vi "Construct.vi"(8 "error in":errorcluster, 9 "status error channel data references":T2 {"specific errors"."timeout" format="%.0x"; "specific errors"."bit timing" format="%.0x"; "specific errors"."long word" format="%.0x"; "specific errors"."parity" format="%.0x"; "specific errors"."gap" format="%.0x"; "receiving" format="%.0x"}, 10 "RT hardware channels":T3[](array[typedef]) {"labels settings for RT"."Label Timestamp Channel Data Reference" format="%.0x"; "labels settings for RT"."Word Initial Raw Value" format="%032.0f"; "labels settings for RT"."Label Disable/Trigger Channel Reference" format="%.0x"; "labels settings for RT"."parameter driver data"."Tx parameter refs" format="%.0x"; "labels settings for RT"."parameter driver data"."Rx block data refs"."Data Reference" format="%.0x"; "labels settings for RT"."SDI" format="%02b"; "labels settings for RT"."label" format="%.0o"}, 11 "ID":string) -> (0 "error out":errorcluster, 3 "Ballard ARINC-429 Rx Execution Unit":refnum<class "Ballard ARINC-429 Rx Execution Unit.lvclass">)   [LabVIEW 2020, in "Ballard ARINC 429 Engine.lvlib" / "Implementation.lvlib" / "Ballard ARINC-429 Rx Execution Unit.lvclass"]
uses:
  Ballard ARINC-429 Rx Execution Unit.lvclass
  Shared/RT Hardware Channel Settings.ctl
  Shared/RT Label Settings.ctl
  Shared/Label.ctl
  Shared/RT Parameters.ctl
  Shared/Parameter Definition.ctl
  Encoding and Decoding/Encoding.ctl
  <vilib>/NI VeriStand/Custom Device API/Block Data Reference.ctl
  <vilib>/NI VeriStand/Custom Device API/Data Reference.ctl
  <vilib>/NI VeriStand/Custom Device API/Custom Device Item Ref.ctl
  Shared/Transfer Type.ctl
  C:/Git/niveristand-ballard-arinc429-custom-device/Source/Custom Device Support/Engine/Implementation/Ballard ARINC-429 Execution Unit/Ballard ARINC-429 Execution Unit.lvclass
  Ballard ARINC-429 Execution Unit/Ballard ARINC-429 Execution Unit.lvclass/Ballard ARINC-429 Execution Unit.ctl
  Ballard ARINC-429 Rx Execution Unit.lvclass/Ballard ARINC-429 Rx Execution Unit.ctl
  Ballard ARINC-429 Execution Unit/Ballard ARINC-429 Execution Unit.lvclass
  C:/Git/niveristand-ballard-arinc429-custom-device/Source/Custom Device Support/Engine/Interfaces/Execution Unit/Execution Unit.lvclass
  C:/Git/niveristand-ballard-arinc429-custom-device/Source/Custom Device Support/Engine/Implementation/Ballard ARINC-429 Rx Execution Unit/Ballard ARINC-429 Rx Execution Unit.lvclass
  Encoding and Decoding/Encoding and Decoding.lvlib
  <vilib>/NI VeriStand/Custom Device API/Custom Device API.lvlib
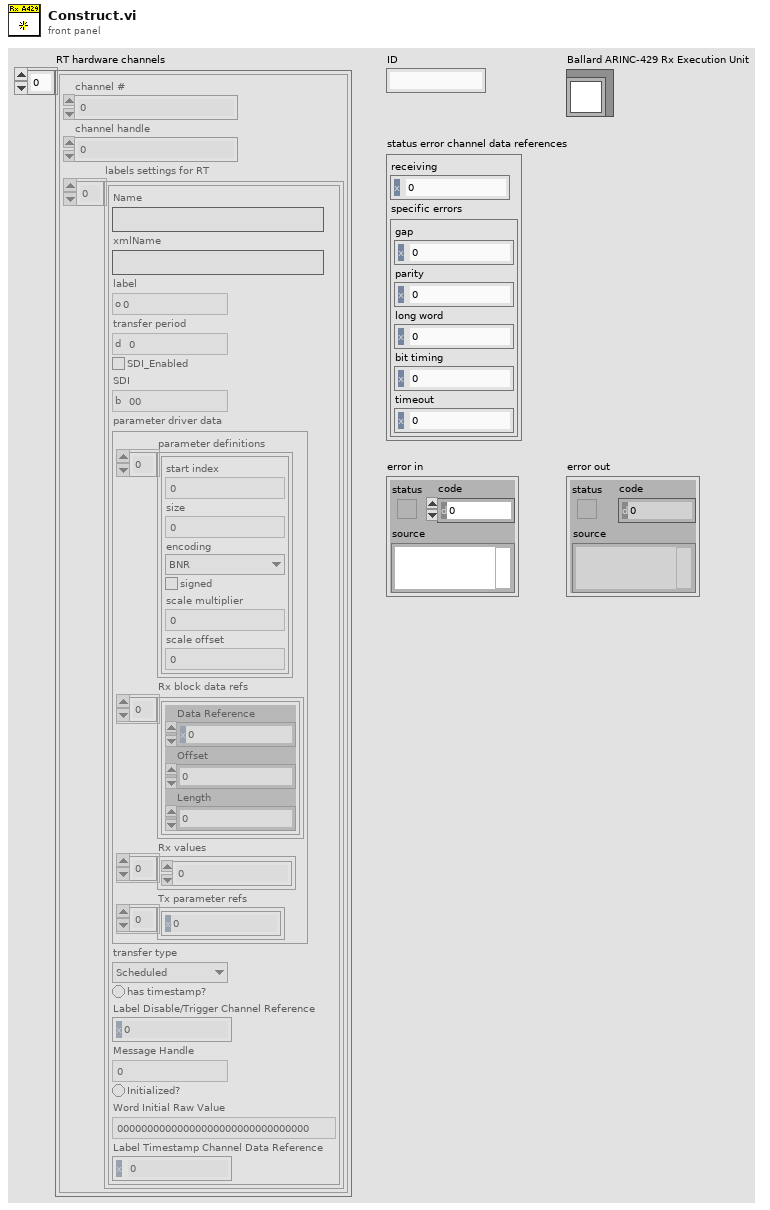
[diagram p1: front panel]
types:
  T1 = typedef "Custom Device API.lvlib/Data Reference.ctl" = i32
  T2 = cluster{"receiving":T1, "specific errors":cluster{"gap":T1, "parity":T1, "long word ":T1, "bit timing":T1, "timeout":T1}}
  T3 = typedef "RT Hardware Channel Settings.ctl" = cluster{"channel #":u16, "channel handle":u64, "labels settings for RT":T4[]}
  T4 = typedef "RT Label Settings.ctl" = cluster{"Name":string, "xmlName":string, "label":T5, "transfer period":u32, "SDI_Enabled":bool, "SDI":u8, "parameter driver data":T6, "transfer type":T11, "has timestamp?":bool, "Label Disable/Trigger Channel Reference":T10, "Message Handle":u64, "Initialized?":bool, "Word Initial Raw Value":u32, "Label Timestamp Channel Data Reference":T1}
  T5 = typedef "Label.ctl" = u8
  T6 = typedef "RT Parameters.ctl" = cluster{"parameter definitions":T7[], "Rx block data refs":T9[], "Rx values":dbl[], "Tx parameter refs":T10[]}
  T7 = typedef "Parameter Definition.ctl" = cluster{"start index":i32, "size":i32, "encoding":T8, "signed":bool, "scale multiplier":dbl, "scale offset":dbl}
  T8 = typedef "Encoding and Decoding.lvlib/Encoding.ctl" = enum16{"BNR", "BCD", "Discrete"}
  T9 = typedef "Custom Device API.lvlib/Block Data Reference.ctl" = cluster{"Data Reference":T1, "Offset":u64, "Length":u64}
  T10 = typedef "Custom Device API.lvlib/Custom Device Item Ref.ctl" = u64
  T11 = typedef "Transfer Type.ctl" = enum16{"Scheduled", "Acyclic", "Block", "Strobe"}
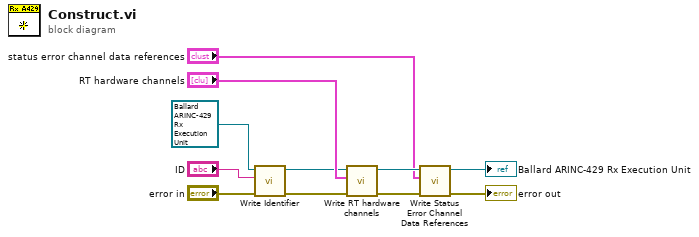
[diagram p0: block diagram]
diagram:
  n1 = call "Write Identifier.vi"("error in (no error)"="error in", "identifier"="ID", "Ballard ARINC-429 Execution Unit in"=refnum<class "Ballard ARINC-429 Rx Execution Unit.lvclass"> refnum ("Ballard ARINC-429 Rx Execution Unit in")) -> ("error out"=w6:errorcluster, "Ballard ARINC-429 Execution Unit out"=w8:refnum<class "Ballard ARINC-429 Rx Execution Unit.lvclass">)  [unwired: 7 in]
  n2 = call "Write RT hardware channels.vi"("error in"=w6, "RT hardware channels"="RT hardware channels", "Ballard ARINC-429 Rx Execution Unit in"=w8) -> ("error out"=w3:errorcluster, "Ballard ARINC-429 Rx Execution Unit out"=w5:refnum<class "Ballard ARINC-429 Rx Execution Unit.lvclass">)  [unwired: 7 in]
  n3 = call "Write Status Error Channel Data References.vi"("error in (no error)"=w3, "status error channel data references"="status error channel data references", "Ballard ARINC-429 Rx Execution Unit in"=w5) -> ("error out"=→"error out":errorcluster, "Ballard ARINC-429 Rx Execution Unit out"=→"Ballard ARINC-429 Rx Execution Unit":refnum<class "Ballard ARINC-429 Rx Execution Unit.lvclass">)  [unwired: 7 in]
